vi "T7 Duct Tape KAG.vi"(7 "incoming":u16[][](array[numeric]), 8 "NumScans requested":u32=1500, 9 "Action":enum16{"Initialize", "Read", "Update"}(ring)) -> (1 "requested":u16[][](array[numeric]))   [LabVIEW 2015]
doc: "Functional Global -- If configuration is such that acquiring all requested samples for a given block dictates reading more samples than requested, then the surplus is stored and appended to the beginning of the subsequent block ~ FIFO."
panel:
  out "overflow":u16[][](array[numeric])
  out "size overflow":i32[](array[numeric])
  out "size requested":i32[](array[numeric])
  out "size incoming":i32[](array[numeric])
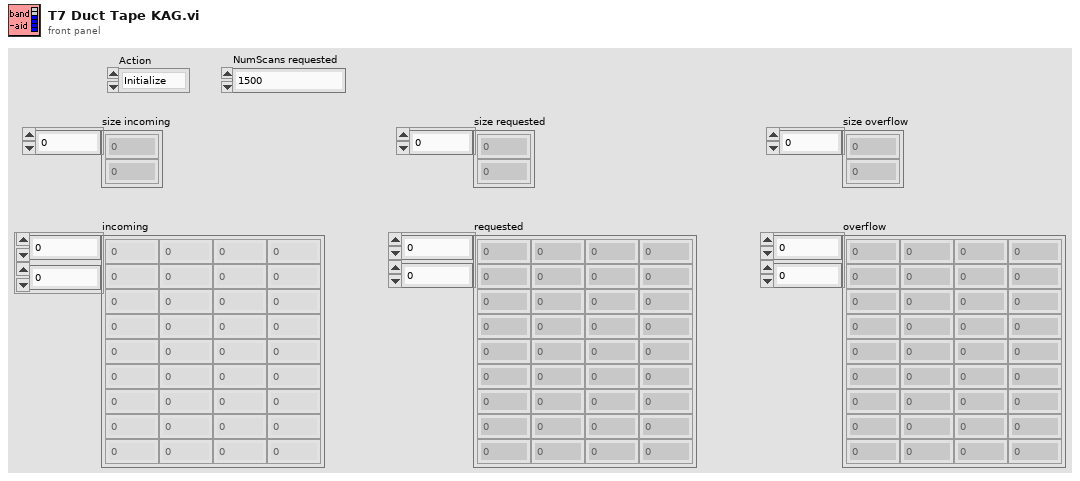
[diagram p1: front panel]
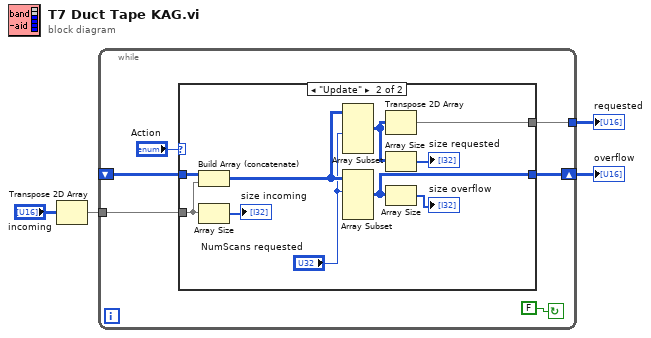
[diagram p0: block diagram]
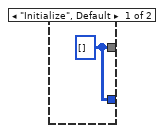
[diagram p2: hidden frame]
diagram:
  n1 = Transpose 2D Array(2D array="incoming") -> (transposed array=w3:u16[][])
  n2 = while {
    shift-right: [w8] -> w1
    shift-left: _ -> [w7]
    tunnel: w3 -> [w6]
    tunnel: [w5] -> w2
    stop <- FALSE continue-if-true
    n3 = case shown="\"Update\"" "Action" {
      tunnel: [w11 w12] -> w8
      tunnel: w7 -> [_ w15]
      tunnel: w6 -> [_ w14]
      tunnel: [w11 w13] -> w5
      frame "Initialize", Default {
        w11 = u16[][] [] ("overflow 2")
      }
      frame "Update" {
        n4 = Build Array (concatenate)(w15, w14) -> (w21:u16[][])
        n5 = Array Size(array=w14) -> (size(s)=→"size incoming":i32[])
        n6 = Array Subset(array=w21, length (row)="NumScans requested") -> (w17:u16[][])  [unwired: 3 in]
        n7 = Array Subset(array=w21, index (row)="NumScans requested") -> (w12:u16[][])  [unwired: 3 in]
        n8 = Transpose 2D Array(2D array=w17) -> (transposed array=w13:u16[][])
        n9 = Array Size(array=w17) -> (size(s)=→"size requested":i32[])
        n10 = Array Size(array=w12) -> (size(s)=→"size overflow":i32[])
      }
    }
  }
  "requested" <- w2
  "overflow" <- w1
